vi "CMC_Homework_08.vi"() -> ()   [LabVIEW 2013]
panel:
  in  "Use System Alert as Tick/Tock?":bool=TRUE
  in  "stop":bool
  in  "Time (sec)":u8(knob) max=60 step=10 scale=0.0..60.0
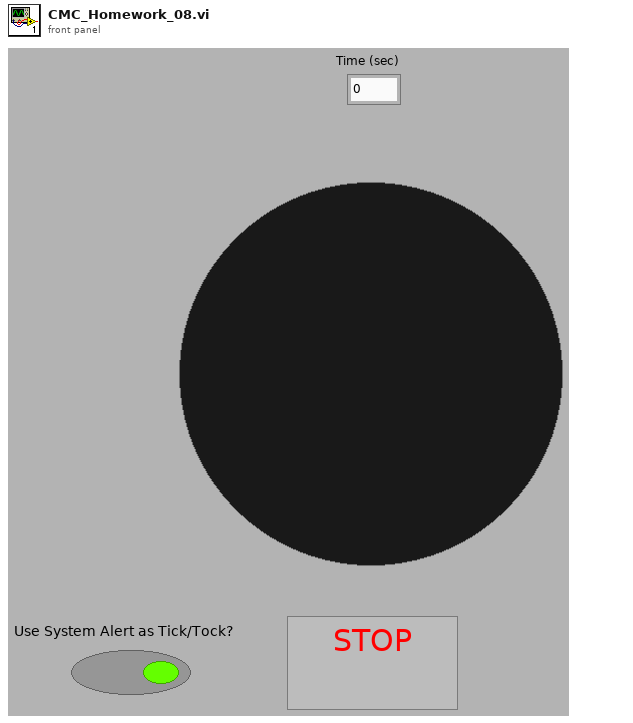
[diagram p1: front panel]
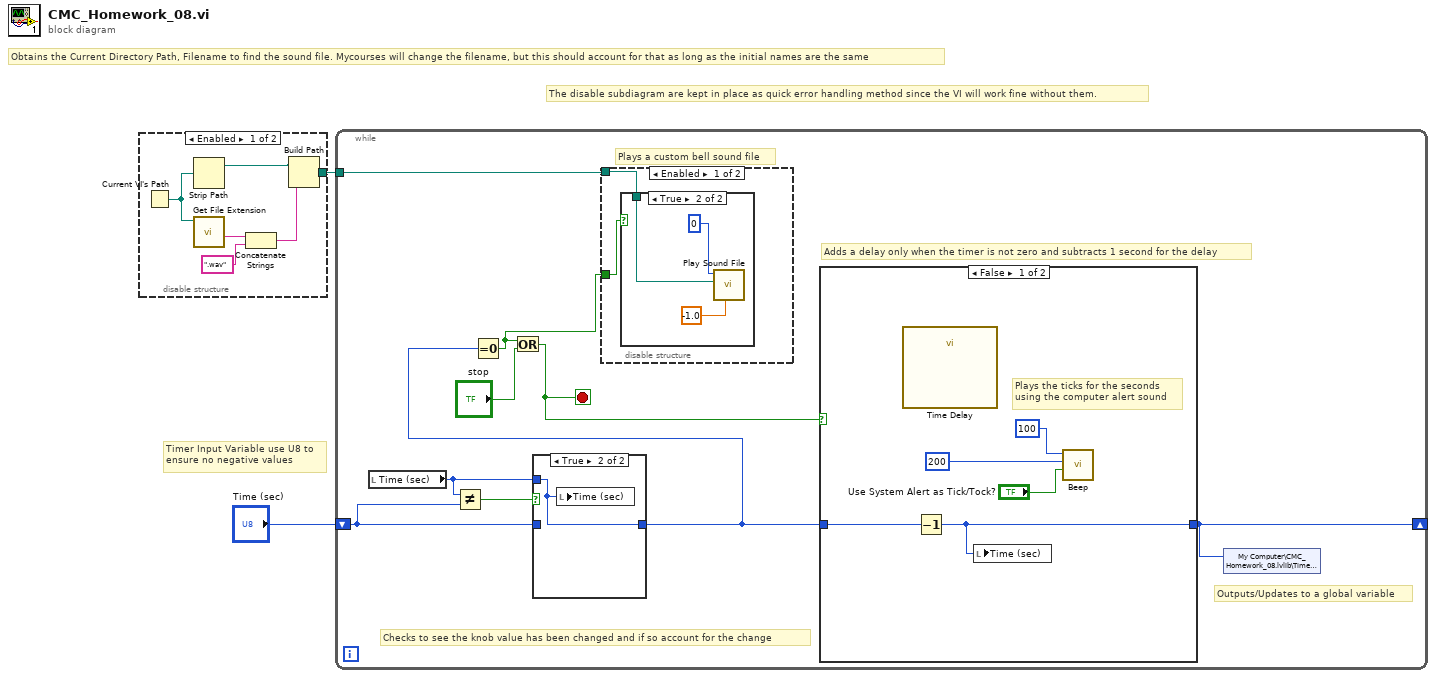
[diagram p0: block diagram]
diagram:
  # "Timer Input Variable use U8 to\nensure no negative values"
  # "The disable subdiagram are kept in place as quick error handling method since the VI will work fine without them."
  # "Obtains the Current Directory Path, Filename to find the sound file. Mycourses will change the filename, but this should account for that as long as the initial names are the same"
  n1 = disable-structure shown="Enabled" {
    disable-tunnel: [w3 _] -> w1
    frame Enabled {
      n2 = Current VI's Path() -> (path=w8:path)
      n3 = Strip Path(path=w8) -> (stripped path=w4:path)  [unwired: 1 out]
      n4 = call <vilib>:"Get File Extension.vi"("file"=w8) -> ("filename without extension"=w7:string)  [unwired: 7 in, 3 out]
      n5 = Concatenate Strings(w7, ".wav") -> (w5:string)
      n6 = Build Path(base path=w4, name or relative path=w5) -> (appended path=w3:path)
    }
    frame Disabled {
    }
  }
  n7 = while {
    shift-right: [w12] -> _
    shift-left: "Time (sec)" -> [w16]
    tunnel: w1 -> [w13]
    stop <- w11 stop-if-true
    # "Outputs/Updates to a global variable"
    # "Adds a delay only when the timer is not zero and subtracts 1 second for the delay"
    # "Checks to see the knob value has been changed and if so account for the change"
    # "Plays a custom bell sound file"
    n8 = local read "Time (sec)"() -> (w17:u8)
    n9 = Not Equal?(x=w17, y=w16) -> (x != y?=w10:bool)
    n10 = case shown="True" w10 {
      tunnel: w17 -> [_ w24]
      tunnel: [w23 w24] -> w9
      tunnel: w16 -> [w23 _]
      frame False {
      }
      frame True {
        n11 = local write "Time (sec)"(w24) -> ()
      }
    }
    n12 = Equal To 0?(x=w9) -> (x = 0?=w15:bool)
    n13 = Or(x=w15, y="stop") -> (x .or. y?=w11:bool)
    n14 = disable-structure shown="Enabled" {
      disable-tunnel: w15 -> [w19 _]
      disable-tunnel: w13 -> [w18 _]
      frame Enabled {
        n15 = case shown="True" w19 {
          tunnel: w18 -> [_ w20]
          frame False {
          }
          frame True {
            n16 = call <vilib>:"Play Sound File.vi"("timeout (sec)"=-1.0, "path"=w20, "device ID"=u32 0) -> ()  [unwired: 7 in, 2 out]
          }
        }
      }
      frame Disabled {
      }
    }
    n17 = case shown="False" w11 {
      tunnel: [w28 w30] -> w12
      tunnel: w9 -> [w29 w30]
      frame False {
        # "Plays the ticks for the seconds\nusing the computer alert sound"
        n18 = call "Time Delay"() -> ()  [unwired: 11 in, 1 out]
        n19 = Decrement(x=w29) -> (x-1=w28:u8)
        n20 = local write "Time (sec)"(w28) -> ()
        n21 = call <vilib>:"Beep.vi"("use system alert? (T)"="Use System Alert as Tick/Tock?", "duration (msec)"=u32 200, "frequency (Hz)"=u32 100) -> ()  [unwired: 9 in]
      }
      frame True {
      }
    }
    n22 = shared-variable "My Computer\\CMC_Homework_08.lvlib\\Time_Left"(w12) -> ()  [unwired: 1 in, 1 out]
  }
